vi "SW_Load_parameter_group_2.vi"(0 "Settings file refnum in":T1, 5 "Researcher name":string, 7 "Parameter group (section)":string, 9 "Default value data in":variant, 11 "error in":errorcluster) -> (4 "Settings file refnum out":T1, 10 "Group (section) cluster data out":variant, 15 "error out":errorcluster)   [LabVIEW 2018, in "Tracker.lvlib"]
uses:
  Tracker.lvlib
  <vilib>/Utility/config.llb/Config Data RefNum.ctl
  <vilib>/Utility/config.llb/NI_LVConfig.lvlib
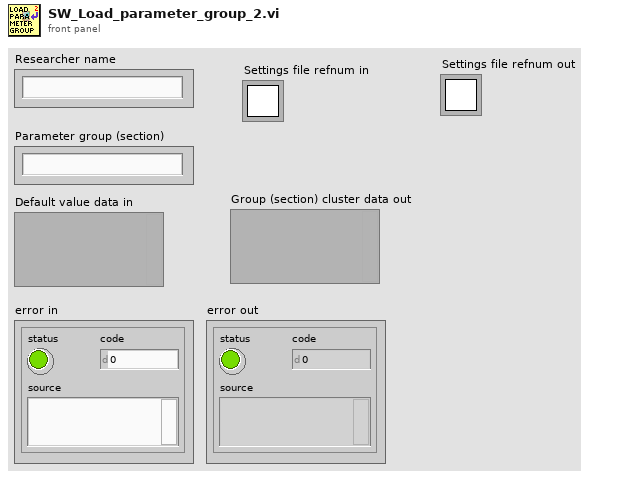
[diagram p1: front panel]
types:
  T1 = typedef "NI_LVConfig.lvlib/Config Data RefNum.ctl" = refnum<k1>
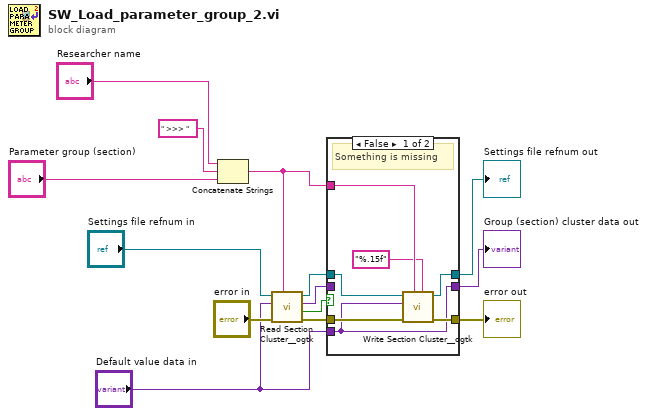
[diagram p0: block diagram]
diagram:
  n1 = Concatenate Strings("Researcher name", " >>> " ("string"), "Parameter group (section)") -> (w2:string)
  n2 = call <userlib>:"Read Section Cluster__ogtk.vi"("section (optional)"=w2, "error in (no error)"="error in", "Section Formatted Cluster Type"="Default value data in", "refnum"="Settings file refnum in") -> ("error out"=w7:errorcluster, "all found?"=w9:bool, "Section Formatted Cluster"=w4:variant, "dup refnum"=w8:T1)  [unwired: 3 in, 1 out]
  n3 = case shown="False" w9 {
    tunnel: w8 -> [w18 w23]
    tunnel: w7 -> [w21 w24]
    tunnel: [w20 w24] -> w5
    tunnel: [w17 w23] -> w6
    tunnel: w4 -> [_ w22]
    tunnel: [w19 w22] -> w3
    tunnel: "Default value data in" -> [w19 _]
    tunnel: w2 -> [w16 _]
    frame False {
      # "Something is missing"
      n4 = call <userlib>:"Write Section Cluster__ogtk.vi"("float number format (optional)"="%.15f", "section (optional)"=w16, "error in (no error)"=w21, "Section Formatted Cluster"=w19, "refnum"=w18) -> ("error out"=w20:errorcluster, "dup refnum"=w17:T1)  [unwired: 5 in]
    }
    frame True {
      # "All data found"
    }
  }
  "error out" <- w5
  "Settings file refnum out" <- w6
  "Group (section) cluster data out" <- w3
